vi "SetVPB.vi"(7 "keep":u8, 8 "error in (no error)":errorcluster, 9 "lines":u32, 10 "range":u32, 11 "board_sel":u32=1) -> (0 "error out":errorcluster)   [LabVIEW 2015, in "ESLSCDLL.lvlib"]
uses:
  ESLSCDLL.lvlib
panel:
  # "Set range for partial binning of FFT"
  # "range 1..5"
  # "lines per range"
  # "1 if range should be kept, 0 then there are a constant"
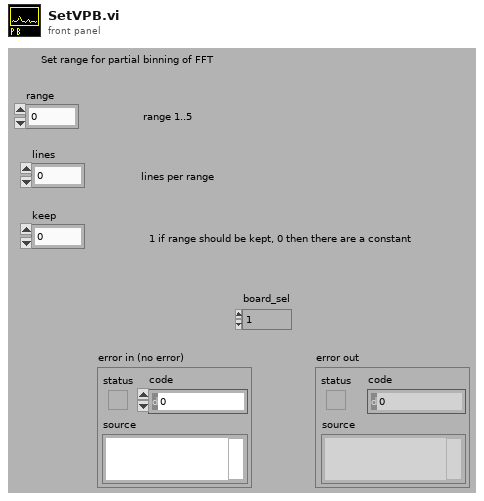
[diagram p1: front panel]
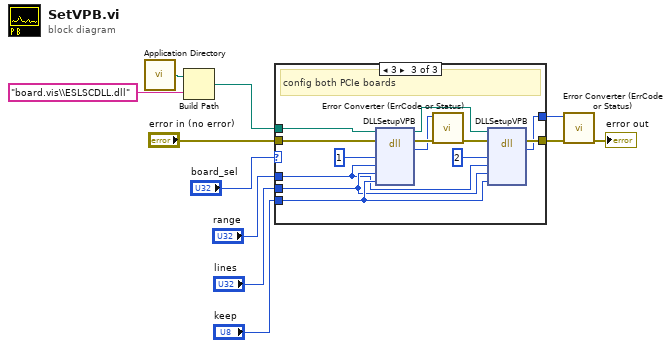
[diagram p0: block diagram]
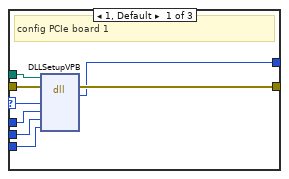
[diagram p2: hidden frame]
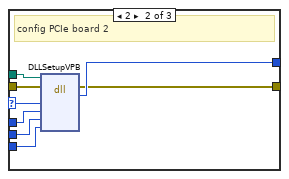
[diagram p3: hidden frame]
diagram:
  n1 = call <vilib>:"Application Directory.vi"() -> ("Application Directory"=w3:path)
  n2 = Build Path(base path=w3, name or relative path="board.vis\\ESLSCDLL.dll") -> (appended path=w1:path)
  n3 = case shown="3" "board_sel" {
    selector: "board_sel" -> [w19 w27 _]
    tunnel: "range" -> [w18 w26 w36]
    tunnel: "lines" -> [w17 w25 w37]
    tunnel: "keep" -> [w16 w24 w38]
    tunnel: [w15 w22 w31] -> w6
    tunnel: "error in (no error)" -> [w14 w21 w35]
    tunnel: [w13 w23 w30] -> w4
    tunnel: w1 -> [w12 w20 w29]
    frame 1, Default {
      # "config PCIe board 1"
      n4 = dll-call lib="C:/ENTW/PCIE/LV64/board.vis/ESLSCDLL.dll" fn="DLLSetupVPB" ("lwlscdll.dll:DLLRsTOREG")(path in=w12, error in=w14, "drv"=w19, "range"=w18, "lines"=w17, "keep"=w16) -> (error out=w15:errorcluster, "es_status_codes"=w13:i32)  [unwired: 5 in, 1 out]
    }
    frame 2 {
      # "config PCIe board 2"
      n5 = dll-call lib="C:/ENTW/PCIE/LV64/board.vis/ESLSCDLL.dll" fn="DLLSetupVPB" ("lwlscdll.dll:DLLRsTOREG")(path in=w20, error in=w21, "drv"=w27, "range"=w26, "lines"=w25, "keep"=w24) -> (error out=w22:errorcluster, "es_status_codes"=w23:i32)  [unwired: 5 in, 1 out]
    }
    frame 3 {
      # "config both PCIe boards"
      n6 = dll-call lib="C:/ENTW/PCIE/LV64/board.vis/ESLSCDLL.dll" fn="DLLSetupVPB" ("lwlscdll.dll:DLLRsTOREG")(path in=w29, error in=w35, "drv"=u32 1, "range"=w36, "lines"=w37, "keep"=w38) -> (path out=w28:path, error out=w34:errorcluster, "es_status_codes"=w33:i32)  [unwired: 5 in]
      n7 = call "Error Converter (ErrCode or Status).vi"("error in (no error)"=w34, "error code"=w33) -> ("error out"=w32:errorcluster)  [unwired: 9 in]
      n8 = dll-call lib="C:/ENTW/PCIE/LV64/board.vis/ESLSCDLL.dll" fn="DLLSetupVPB" ("lwlscdll.dll:DLLRsTOREG")(path in=w28, error in=w32, "drv"=u32 2, "range"=w36, "lines"=w37, "keep"=w38) -> (error out=w31:errorcluster, "es_status_codes"=w30:i32)  [unwired: 5 in, 1 out]
    }
  }
  n9 = call "Error Converter (ErrCode or Status).vi"("error in (no error)"=w6, "error code"=w4) -> ("error out"=→"error out":errorcluster)  [unwired: 9 in]
